vi "1Cx2x3-Small RC.vi"() -> ()   [LabVIEW 2011]
uses:
  2-RIO/2 Globals/2 Global.vi
panel:
  in  "Sense Data Source":enum16{"Overhead Camera", "Simulation"}(ring)
  # "this is the parent VI under which \nthe Small RC Boat's sensors, RIO and OCU run."
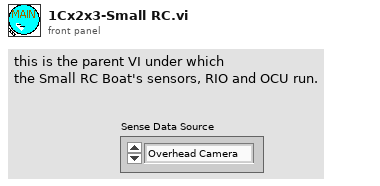
[diagram p1: front panel]
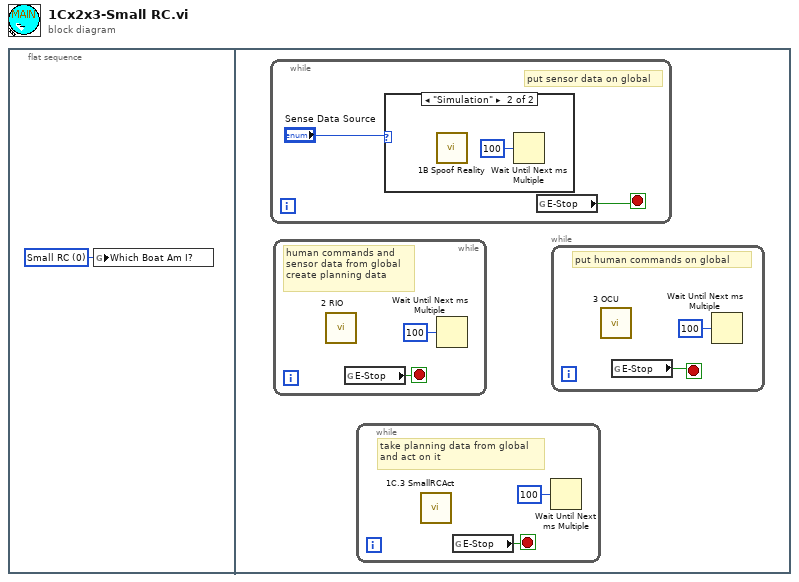
[diagram p0: block diagram]
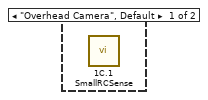
[diagram p2: hidden frame]
diagram:
  n1 = flat-sequence {
    frame #0 {
      w1 = u16 0 items=["Small RC", "Large RC", "Final Boat", "Simulator"] ("Which Boat Am I?")
      n2 = global write "2 Global.vi" "Which Boat Am I?"(w1) -> ()
    }
    frame #1 {
      n3 = while {
        stop <- w8 stop-if-true
        # "put sensor data on global"
        n4 = case shown="\"Simulation\"" "Sense Data Source" {
          frame "Overhead Camera", Default {
            n5 = call "1C.1 SmallRCSense.vi"() -> ()  [unwired: 6 in, 6 out]
          }
          frame "Simulation" {
            n6 = call "1B Spoof Reality.vi"() -> ()  [unwired: 6 in, 6 out]
            n7 = Wait Until Next ms Multiple(millisecond multiple=u32 100) -> ()  [unwired: 1 out]
          }
        }
        n8 = global read "2 Global.vi" "E-Stop"() -> (w8:bool)
      }
      n9 = while {
        stop <- w4 stop-if-true
        # "human commands and \nsensor data from global\ncreate planning data"
        n10 = call "2 RIO.vi"() -> ()  [unwired: 12 in]
        n11 = global read "2 Global.vi" "E-Stop"() -> (w4:bool)
        n12 = Wait Until Next ms Multiple(millisecond multiple=u32 100) -> ()  [unwired: 1 out]
      }
      n13 = while {
        stop <- w6 stop-if-true
        # "take planning data from global\nand act on it"
        n14 = call "1C.3 SmallRCAct.vi"() -> ()  [unwired: 12 in]
        n15 = global read "2 Global.vi" "E-Stop"() -> (w6:bool)
        n16 = Wait Until Next ms Multiple(millisecond multiple=u32 100) -> ()  [unwired: 1 out]
      }
      n17 = while {
        stop <- w2 stop-if-true
        # "put human commands on global"
        n18 = call "3 OCU.vi"() -> ()  [unwired: 12 in]
        n19 = global read "2 Global.vi" "E-Stop"() -> (w2:bool)
        n20 = Wait Until Next ms Multiple(millisecond multiple=u32 100) -> ()  [unwired: 1 out]
      }
    }
  }
